vi "HandleRightClickMenuOption.vi"(0 "reference":refnum<class "StateDiagramGraph.lvclass">, 1 "MenuOption":string, 2 "graphics":refnum<class "Graphics.lvclass">, 3 "grid":refnum<class "Grid.lvclass">, 4 "point":T1 {"y" format="%.2f"; "x" format="%.2f"}, 5 "error in (no error)":errorcluster) -> (14 "reference out":refnum<class "StateDiagramGraph.lvclass">, 15 "Cancel":bool, 19 "error out":errorcluster)   [LabVIEW 2014, in "StateDiagramGraph.lvclass"]
doc: "HandleRightClickMenuOption"
uses:
  <resource>/Framework/Providers/Open_GDS/UML/StateDiagramGraph_class/StateDiagramGraph.lvclass
  <resource>/Framework/Providers/Open_GDS/UML/Graphics_class/Graphics.lvclass
  <resource>/Framework/Providers/Open_GDS/UML/Grid_class/Grid.lvclass
  <resource>/Framework/Providers/Open_GDS/UML/General/Point/Point Point2D.ctl
  <resource>/Framework/Providers/Open_GDS/UML/ReversedEngineering/private/ReversedEngineering StateDiagramReverseOptions.ctl
  <resource>/Framework/Providers/Open_GDS/UML/ReversedEngineering/private/ReversedEngineering StateDiagramSerachActions.ctl
  <resource>/Framework/Providers/Open_GDS/UML/ReversedEngineering/ReversedEngineering StateAnalyseVIAction.ctl
  <resource>/Framework/Providers/Open_GDS/UML/ReversedEngineering/private/ReversedEngineering StateDiagramCommentSearchType.ctl
  <resource>/Framework/Providers/Open_GDS/UML/UMLEditor/UMLEditor BusyDialogAction.ctl
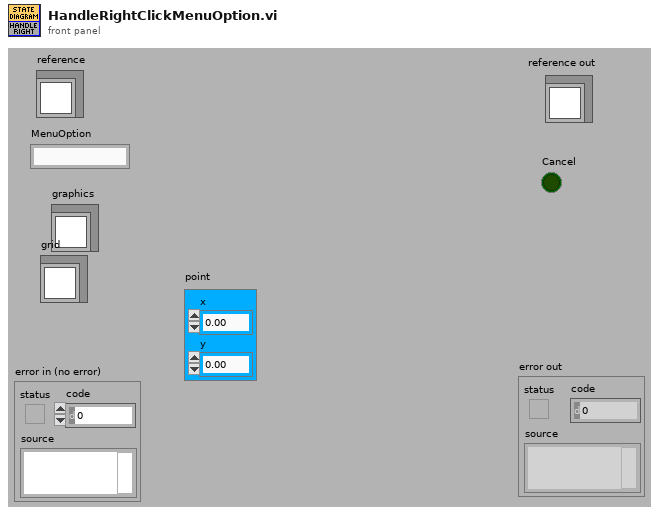
[diagram p1: front panel]
types:
  T1 = typedef "Point Point2D.ctl" = cluster{"x":dbl, "y":dbl}
  T2 = typedef "ReversedEngineering StateDiagramReverseOptions.ctl" = cluster{"Clear All Current States":bool, "UseMenuItem":bool, "InsertArrayQueuedElementsVI":string, "Add Actions":bool, "StateDiagramSerachActions":T3, "AddCaseCommentsAsActions":bool, "IgnoreStatesNotUsed":bool, "CommentsSerachActions":T5, "TransitionMode":enum16{"Add to current transtion text", "Replace transition text"}, "ActionMode":enum16{"Add to current action text", "Replace action text"}}
  T3 = typedef "ReversedEngineering StateDiagramSerachActions.ctl" = cluster{"Action":T4, "VINames":string[], "LimitActions(VIs)":i32}
  T4 = typedef "ReversedEngineering StateAnalyseVIAction.ctl" = enum16{"OnlyTheseVIs", "NotTheseVIs"}
  T5 = typedef "ReversedEngineering StateDiagramCommentSearchType.ctl" = cluster{"MinimumTextLength":i32, "OnlyTopLeftComment":bool, "CommentPrefix":string}
  T6 = typedef "UMLEditor BusyDialogAction.ctl" = enum16{"Initialize", "Open(VIs)", "Open(i)", "Send_I-Value", "SendStatusMessage", "GetBusyDialogStatus", "Close", "Quit"}
  T7 = typedef "StateDiagramGraph.lvclass/ObjectAttributes.ctl" = cluster{"Base class":T8, "StateDiagramData":T9}
  T8 = typedef "Graph.lvclass/ObjectAttributes.ctl" = cluster{"nodes":refnum<class "AbstractNode.lvclass">[], "edges":refnum<class "AbstractEdge.lvclass">[], "nodesToBeRemoved":refnum<class "AbstractNode.lvclass">[], "edgesToBeRemoved":refnum<class "AbstractEdge.lvclass">[], "needsLayout":bool, "LayoutNodes":refnum<class "AbstractNode.lvclass">[]}
  T9 = typedef "StateDiagramGraph.lvclass/StateDiagramData.ctl" = cluster{"VI-Path":path, "ShowOption":T10}
  T10 = typedef "StateDiagramGraph.lvclass/ViPathShowOption.ctl" = enum16{"Don't Show", "Show Relative Path", "Show Absolute Path"}
  T11 = typedef "ReversedEngineering StateMachineStateInfo.ctl" = cluster{"State":string, "TransitionStates":string[], "Actions":string[], "Comments":string[], "TransactionText":string[]}
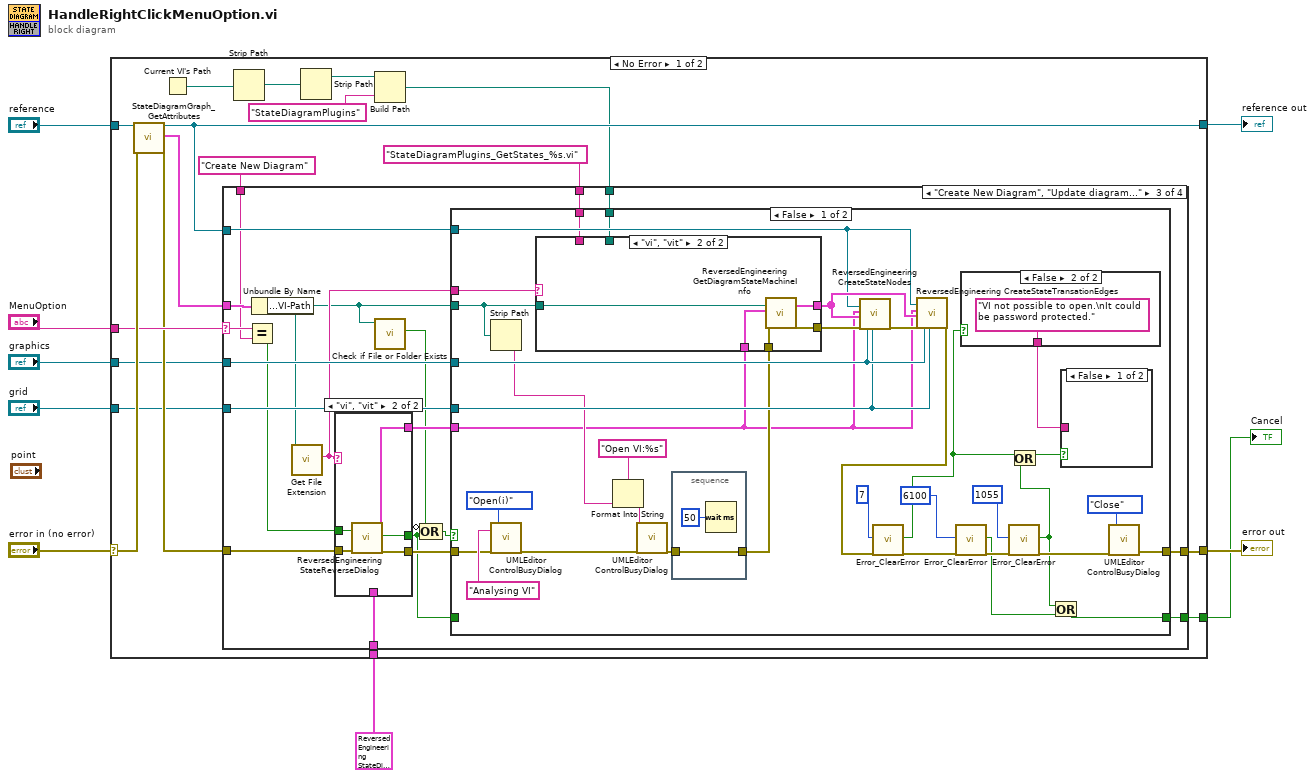
[diagram p0: block diagram]
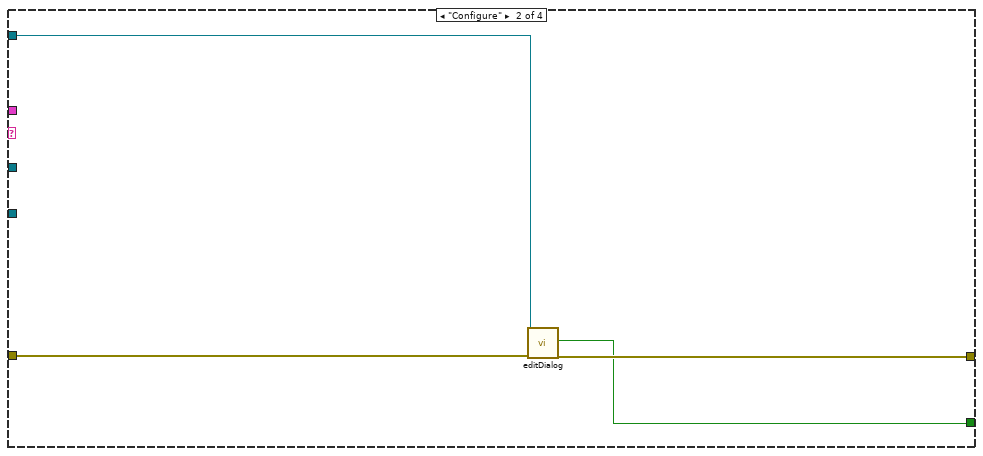
[diagram p3: hidden frame]
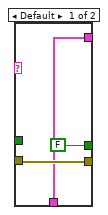
[diagram p4: hidden frame]
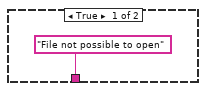
[diagram p5: hidden frame]
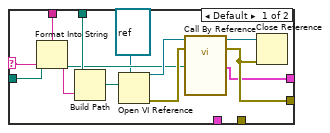
[diagram p6: hidden frame]
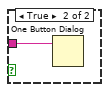
[diagram p7: hidden frame]
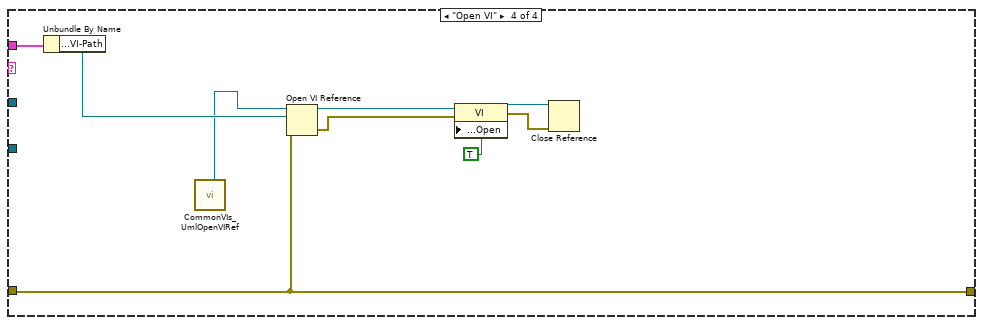
[diagram p9: hidden frame]
diagram:
  n1 = case shown="No Error" "error in (no error)" {
    selector: "error in (no error)" -> [w27 w129]
    tunnel: "reference" -> [w26 w130]
    tunnel: [w22 w129] -> w7
    tunnel: [w23 w130] -> w6
    tunnel: "MenuOption" -> [w25 _]
    tunnel: "graphics" -> [w20 _]
    tunnel: "grid" -> [w19 _]
    tunnel: [w18 _] -> w2
    tunnel: T2 {"Clear All Current States"=TRUE, "UseMenuItem"=FALSE, "InsertArrayQueuedElementsVI"="", "Add Actions"=TRUE, "StateDiagramSerachActions"={"Action"=enum."OnlyTheseVIs", "VINames"=[], "LimitActions(VIs)"=0}, "AddCaseCommentsAsActions"=FALSE, "IgnoreStatesNotUsed"=FALSE, "CommentsSerachActions"={"MinimumTextLength"=0, "OnlyTopLeftComment"=FALSE, "CommentPrefix"=""}, "TransitionMode"=enum."Add to current transtion text", "ActionMode"=enum."Add to current action text"} ("StateDiagramReverseOptions") -> [w10 _]
    frame No Error {
      n2 = call <resource>:"StateDiagramGraph_GetAttributes.vi"("reference in"=w26, "error in (no error)"=w27) -> ("reference out"=w23:refnum<class "StateDiagramGraph.lvclass">, "Attributes"=w21:T7, "error out"=w24:errorcluster)  [unwired: 15 out]
      n3 = Current VI's Path() -> (path=w16:path)
      n4 = Strip Path(path=w16) -> (stripped path=w15:path)  [unwired: 1 out]
      n5 = Strip Path(path=w15) -> (stripped path=w13:path)  [unwired: 1 out]
      n6 = Build Path(base path=w13, name or relative path="StateDiagramPlugins") -> (appended path=w12:path)
      n7 = case shown="\"Create New Diagram\", \"Update diagram...\"" w25 {
        selector: w25 -> [_ _ w44 _]
        tunnel: w24 -> [w28 w32 w47 w121]
        tunnel: w23 -> [_ w31 w51 _]
        tunnel: [w28 w30 w48 w121] -> w22
        tunnel: w21 -> [_ _ w52 w123]
        tunnel: w20 -> [_ _ w50 _]
        tunnel: w19 -> [_ _ w49 _]
        tunnel: [_ w29 w40 _] -> w18
        tunnel: "Create New Diagram" ("y") -> [_ _ w43 _]
        tunnel: w12 -> [_ _ w38 _]
        tunnel: "StateDiagramPlugins_GetStates_%s.vi" ("y") -> [_ _ w37 _]
        tunnel: w10 -> [_ _ w33 _]
        frame "False", Default {
        }
        frame "Configure" {
          n8 = call-dynamic "editDialog.vi"("reference"=w31, "error in (no error)"=w32) -> ("cancel"=w29:bool, "error out"=w30:errorcluster)  [unwired: 15 in, 1 out]
        }
        frame "Create New Diagram", "Update diagram..." {
          n9 = Equal?(x=w44, y=w43) -> (x = y?=w42:bool)
          n10 = Unbundle By Name(w52) -> ("StateDiagramData.VI-Path"=w36:path)
          n11 = call <vilib>:"Get File Extension.vi"("file"=w36) -> ("lowercase file extension"=w39:string)  [unwired: 1 in, 9 out]
          n12 = case shown="\"vi\", \"vit\"" w39 {
            tunnel: w47 -> [w55 w60]
            tunnel: [w55 w59] -> w46
            tunnel: [w53 w58] -> w45
            tunnel: w42 -> [_ w57]
            tunnel: [FALSE ("Cancel") w56] -> w41
            tunnel: w33 -> [w53 _]
            frame Default {
            }
            frame "vi", "vit" {
              n13 = call <resource>:"ReversedEngineering StateReverseDialog.vi"("error in (no error)"=w60, "NewDiagram"=w57) -> ("StateDiagramReverseOptions"=w58:T2, "Cancel"=w56:bool, "error out"=w59:errorcluster)  [unwired: 15 out]
            }
          }
          n14 = call <vilib>:"Check if File or Folder Exists.vi"("path"=w36) -> ("file or folder exists?"=w34:bool)  [unwired: 1 in, 9 out]
          n15 = Compound Arithmetic op=OR(invert w34, w41) -> (w35:bool)
          n16 = case shown="False" w35 {
            tunnel: w36 -> [w81 _]
            tunnel: w51 -> [w93 _]
            tunnel: w50 -> [w92 _]
            tunnel: w49 -> [w91 _]
            tunnel: [w84 w119] -> w48
            tunnel: w46 -> [w86 w119]
            tunnel: w45 -> [w61 _]
            tunnel: w41 -> [_ w118]
            tunnel: [w73 w118] -> w40
            tunnel: w39 -> [w71 _]
            tunnel: w38 -> [w70 _]
            tunnel: w37 -> [w69 _]
            frame False {
              n17 = Strip Path(path=w81) -> (name=w62:string)  [unwired: 1 out]
              n18 = call <resource>:"UMLEditor ControlBusyDialog.vi"("Title/StatusText"="Analysing VI", "error in (no error)"=w86, "Action(SendStatusMessage)"=UMLEditor_BusyDialogAction."Open(i)" ("Action")) -> ("error out"=w83:errorcluster)  [unwired: 1 in, 15 out]
              n19 = Format Into String(format string="Open VI:%s", w62) -> (resulting string=w79:string)  [unwired: 2 in, 1 out]
              n20 = call <resource>:"UMLEditor ControlBusyDialog.vi"("Title/StatusText"=w79, "error in (no error)"=w83) -> ("error out"=w82:errorcluster)  [unwired: 2 in, 15 out]
              n21 = stacked-sequence {
                tunnel: [w117] -> w87
                tunnel: w82 -> [w117]
                frame #0 {
                  n22 = Wait (ms)(milliseconds to wait=u32 50) -> ()  [unwired: 1 out]
                }
              }
              n23 = case shown="\"vi\", \"vit\"" w71 {
                selector: w71 -> [w106 _]
                tunnel: [w100 w114] -> w95
                tunnel: [w98 w113] -> w94
                tunnel: w61 -> [_ w112]
                tunnel: w87 -> [_ w111]
                tunnel: w81 -> [w102 w110]
                tunnel: w70 -> [w108 _]
                tunnel: w69 -> [w107 _]
                frame Default {
                  n24 = Format Into String(format string=w107, w106) -> (resulting string=w105:string)  [unwired: 2 in, 1 out]
                  n25 = Build Path(base path=w108, name or relative path=w105) -> (appended path=w109:path)
                  n26 = Open VI Reference(type specifier VI Refnum (for type only)=refnum<vi> refnum, vi path=w109) -> (vi reference=w104:refnum<vi>, error out=w103:errorcluster)  [unwired: 1 in, 3 out]
                  n27 = call-by-ref "?"(reference=w104, error in=w103, "Path"=w102) -> (reference out=w101:refnum<vi>, error out=w100:errorcluster, "States"=w98:T11[])  [unwired: 17 in, 1 out]
                  n28 = Close Reference(reference=w101, error in (no error)=w100) -> ()  [unwired: 1 out]
                }
                frame "vi", "vit" {
                  n29 = call <resource>:"ReversedEngineering GetDiagramStateMachineInfo.vi"("Path"=w110, "StateDiagramReverseOptions"=w112, "error in (no error)"=w111) -> ("States"=w113:T11[], "error out"=w114:errorcluster)  [unwired: 15 out]
                }
              }
              n30 = call <resource>:"ReversedEngineering CreateStateNodes.vi"("GraphRefToAddNodesTo"=w93, "StateDiagramReverseOptions"=w61, "States"=w94, "error in (no error)"=w95, "graphics"=w92, "grid"=w91) -> ("error out"=w90:errorcluster)  [unwired: 13 out]
              n31 = call <resource>:"ReversedEngineering CreateStateTransationEdges.vi"("GraphRefToAddNodesTo"=w93, "StateDiagramReverseOptions"=w61, "States"=w94, "error in (no error)"=w90, "graphics"=w92, "grid"=w91) -> ("error out"=w67:errorcluster)  [unwired: 13 out]
              n32 = call <resource>:"Error_ClearError.vi"("code"=7, "error in (no error)"=w67) -> ("Cleared?"=w63:bool, "error out"=w68:errorcluster)  [unwired: 3 in, 13 out]
              n33 = call <resource>:"Error_ClearError.vi"("code"=6100, "error in (no error)"=w68) -> ("Cleared?"=w74:bool, "error out"=w77:errorcluster)  [unwired: 3 in, 13 out]
              n34 = case shown="False" w63 {
                tunnel: ["File not possible to open" ("message") "VI not possible to open.\nIt could be password protected." ("message")] -> w72
                frame True {
                }
                frame False {
                }
              }
              n35 = call <resource>:"Error_ClearError.vi"("code"=1055, "error in (no error)"=w77) -> ("Cleared?"=w64:bool, "error out"=w75:errorcluster)  [unwired: 3 in, 13 out]
              n36 = Or(x=w63, y=w64) -> (x .or. y?=w65:bool)
              n37 = Or(x=w64, y=w74) -> (x .or. y?=w73:bool)
              n38 = case shown="False" w65 {
                tunnel: w72 -> [_ w115]
                frame False {
                }
                frame True {
                  n39 = One Button Dialog(message=w115) -> ()  [unwired: 2 out]
                }
              }
              n40 = call <resource>:"UMLEditor ControlBusyDialog.vi"("error in (no error)"=w75, "Action(SendStatusMessage)"=UMLEditor_BusyDialogAction."Close") -> ("error out"=w84:errorcluster)  [unwired: 2 in, 15 out]
            }
            frame True {
            }
          }
        }
        frame "Open VI" {
          n41 = Unbundle By Name(w123) -> ("StateDiagramData.VI-Path"=w122:path)
          n42 = call <resource>:"CommonVIs_UmlOpenVIRef.vi"() -> ("AppRefOut"=w120:refnum<vi>)  [unwired: 4 in, 7 out]
          n43 = Open VI Reference(application reference (local)=w120, vi path=w122, error in (no error)=w121) -> (vi reference=w128:refnum<vi>, error out=w124:errorcluster)  [unwired: 3 out]
          n44 = property class="VI"(reference=w128, error in=w124, "Front Panel Window:Open"=TRUE) -> (reference out=w126:refnum<vi>, error out=w125:errorcluster)
          n45 = Close Reference(reference=w126, error in (no error)=w125) -> ()  [unwired: 1 out]
        }
      }
    }
    frame Error {
    }
  }
  "reference out" <- w6
  "error out" <- w7
  "Cancel" <- w2
